vi "Read Bytes.vi"(8 "error in (no error)":errorcluster {"code" format="%.0x"}, 9 "BufferSize":i64=2048, 11 "instrument handle":refnum<k15>) -> (0 "error out":errorcluster {"code" format="%.0x"}, 1 "ReturnCount":i64, 2 "Buffer":u32[](array[numeric]), 3 "instrument handle out":refnum<k15>)   [LabVIEW 2020, in "Keysight DAQ970.lvlib"]
doc: "Reads a complete response from the instrument."
uses:
  Keysight DAQ970.lvlib
  KtDAQ970.dll
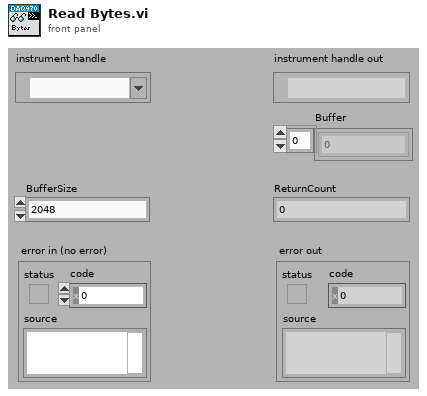
[diagram p1: front panel]
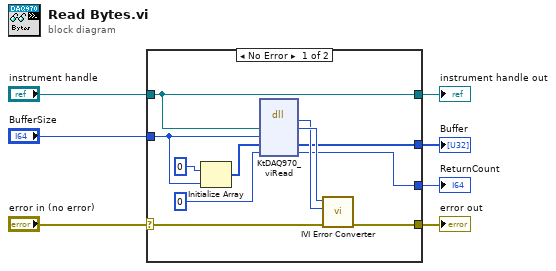
[diagram p0: block diagram]
diagram:
  n1 = case shown="No Error" "error in (no error)" {
    selector: "error in (no error)" -> [w16 w20]
    tunnel: [w15 w20] -> w7
    tunnel: "instrument handle" -> [w11 w19]
    tunnel: "BufferSize" -> [w10 _]
    tunnel: [w14 _] -> w1
    tunnel: [w12 _] -> w3
    tunnel: [w11 w19] -> w2
    frame No Error {
      n2 = Initialize Array(i64 0 ("ReturnCount"), w10) -> (w9:i64[])
      n3 = dll-call lib="KtDAQ970**.dll" fn="KtDAQ970_viRead"("Vi"=w11, "BufferSize"=w10, "Buffer"=w9, "ReturnCount"=i64 0) -> ("return type"=w17:i32, "Vi"=w18:u32, "Buffer"=w14:u32[], "ReturnCount"=w12:i64)  [unwired: 4 in, 2 out]
      n4 = call "IVI Error Converter.vi"("error in (no error)"=w16, "IVI error code (0)"=w17, "instrument handle"=w18) -> ("error out"=w15:errorcluster)  [unwired: 7 in, 1 out]
    }
    frame Error {
    }
  }
  "error out" <- w7
  "instrument handle out" <- w2
  "ReturnCount" <- w3
  "Buffer" <- w1
